vi "Day 15-1.vi"() -> ()   [LabVIEW 2019, in "Day 15.lvlib"]
uses:
  Day 15.lvlib
  Controls/Coordenate.ctl
panel:
  out "Min Distance Last Point":u32
  out "Min Distance Matrix":u32[][](array[numeric])
  out "Array":u8[][](array[numeric])
  in  "String":string="1163751742\n1381373672\n2136511328\n3694931569\n7463417111\n1319128137\n1359912421\n3125421639\n1293138521\n2311944581"
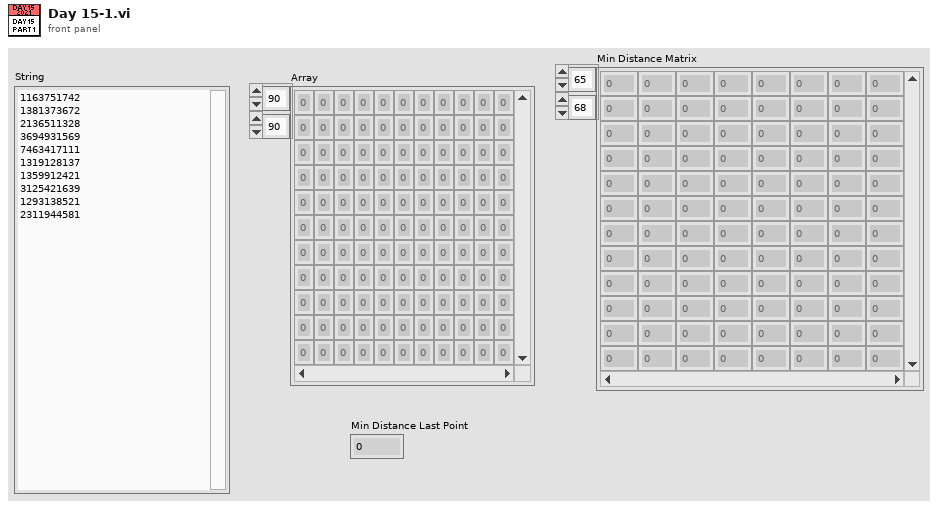
[diagram p1: front panel]
types:
  T1 = typedef "Day 15.lvlib/Coordenate.ctl" = cluster{"Row":i32, "Column":i32}
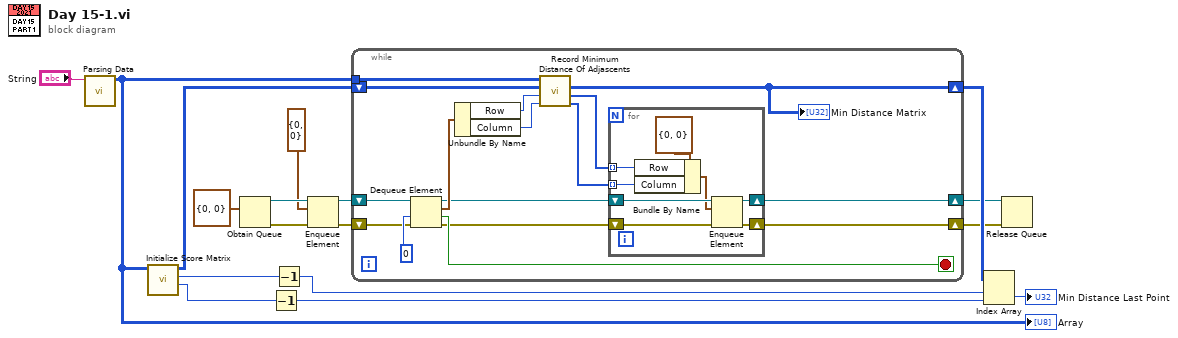
[diagram p0: block diagram]
diagram:
  n1 = call "Parsing Data.vi"("String"="String") -> ("Array"=w12:u8[][])  [unwired: 10 in]
  "Array" <- w12
  n2 = call "Initialize Score Matrix.vi"("Data Matrix"=w12) -> ("Columns"=w15:i32, "Rows"=w16:i32, "Score Matrix"=w11:u32[][])  [unwired: 8 in]
  n3 = Obtain Queue(element data type=T1 {"Row"=0, "Column"=0} ("Coordenate")) -> (queue out=w7:refnum<queue>, error out=w5:errorcluster)  [unwired: 4 in, 1 out]
  n4 = Decrement(x=w15) -> (x-1=w13:i32)
  n5 = Decrement(x=w16) -> (x-1=w14:i32)
  n6 = Enqueue Element(queue=w7, element=T1 {"Row"=0, "Column"=0}, error in (no error)=w5) -> (queue out=w4:refnum<queue>, error out=w3:errorcluster)  [unwired: 1 in, 1 out]
  n7 = while {
    tunnel: w12 -> [w33]
    shift-right: [w31] -> w10
    shift-left: w11 -> [w32]
    shift-right: [w19] -> w2
    shift-left: w4 -> [w30]
    shift-right: [w18] -> w1
    shift-left: w3 -> [w27]
    stop <- w29 stop-if-true
    n8 = Dequeue Element(queue=w30, timeout in ms (-1)=0, error in (no error)=w27) -> (queue out=w21:refnum<queue>, element=w26:T1, timed out?=w29:bool, error out=w20:errorcluster)
    n9 = Unbundle By Name(w26) -> ("Row"=w25:i32, "Column"=w24:i32)
    n10 = call "Record Minimum Distance Of Adjascents.vi"("Column In"=w24, "Row In"=w25, "Minimum Distance Matrix In"=w32, "Data Matrix"=w33) -> ("Columns Out"=w22:i32[], "Rows Out"=w23:i32[], "Minimum Distance Matrix Out"=w31:u32[][])  [unwired: 5 in]
    "Min Distance Matrix" <- w31
    n11 = for {
      tunnel: w23 -> [w40] mode=indexing
      tunnel: w22 -> [w39] mode=indexing
      shift-right: [w36] -> w19
      shift-left: w21 -> [w37]
      shift-right: [w35] -> w18
      shift-left: w20 -> [w38]
      n12 = Bundle By Name(cluster=T1 {"Row"=0, "Column"=0} ("Coordenate"), "Row"=w40, "Column"=w39) -> (w34:T1)
      n13 = Enqueue Element(queue=w37, element=w34, error in (no error)=w38) -> (queue out=w36:refnum<queue>, error out=w35:errorcluster)  [unwired: 1 in, 1 out]
    }
  }
  n14 = Index Array(array=w10, index (row)=w14, index (col)=w13) -> (element=→"Min Distance Last Point":u32)
  n15 = Release Queue(queue=w2, error in (no error)=w1) -> ()  [unwired: 1 in, 3 out]
